vi "Hot Goal Detection - Image Compare.vi"(0 "Image In":T1, 7 "error in":errorcluster) -> (20 "Image Out":T1, 21 "Matches (tape)":T2(array[cluster]) {"Bounding Box"."y" format="%.2f"; "Bounding Box"."x" format="%.2f"; "Position"."y" format="%.2f"; "Position"."x" format="%.2f"; "Score" format="%.2f"; "Scale" format="%.2f"; "Angle" format="%.2f"}, 27 "error out":errorcluster)   [LabVIEW 2013]
uses:
  <vilib>/vision/Image Controls.llb/IMAQ Image.ctl
  <vilib>/vision/NI_Vision_Development_Module.lvlib
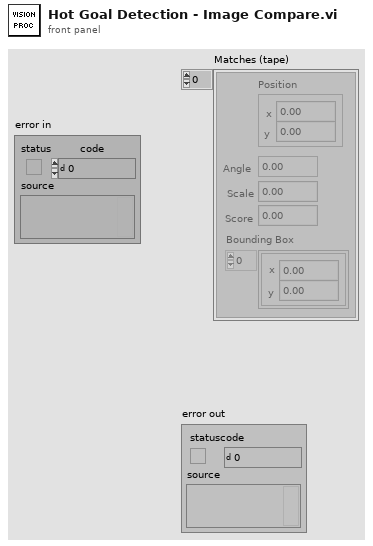
[diagram p1: front panel]
types:
  T1 = typedef "IMAQ Image.ctl" = refnum<image>
  T2 = cluster{"Position":cluster{"x":sgl, "y":sgl}, "Angle":sgl, "Scale":sgl, "Score":sgl, "Bounding Box":cluster{"x":sgl, "y":sgl}[]}[]
  T3 = typedef "Image Type" = u32
  T4 = cluster{"Global Rectangle":i32[], "Contours":cluster{"ID":enum32{"External", "Internal"}, "Type":u32, "Coordinates":i32[]}[]}
  T5 = cluster{"Brightness":sgl, "Contrast":sgl, "Gamma":sgl}
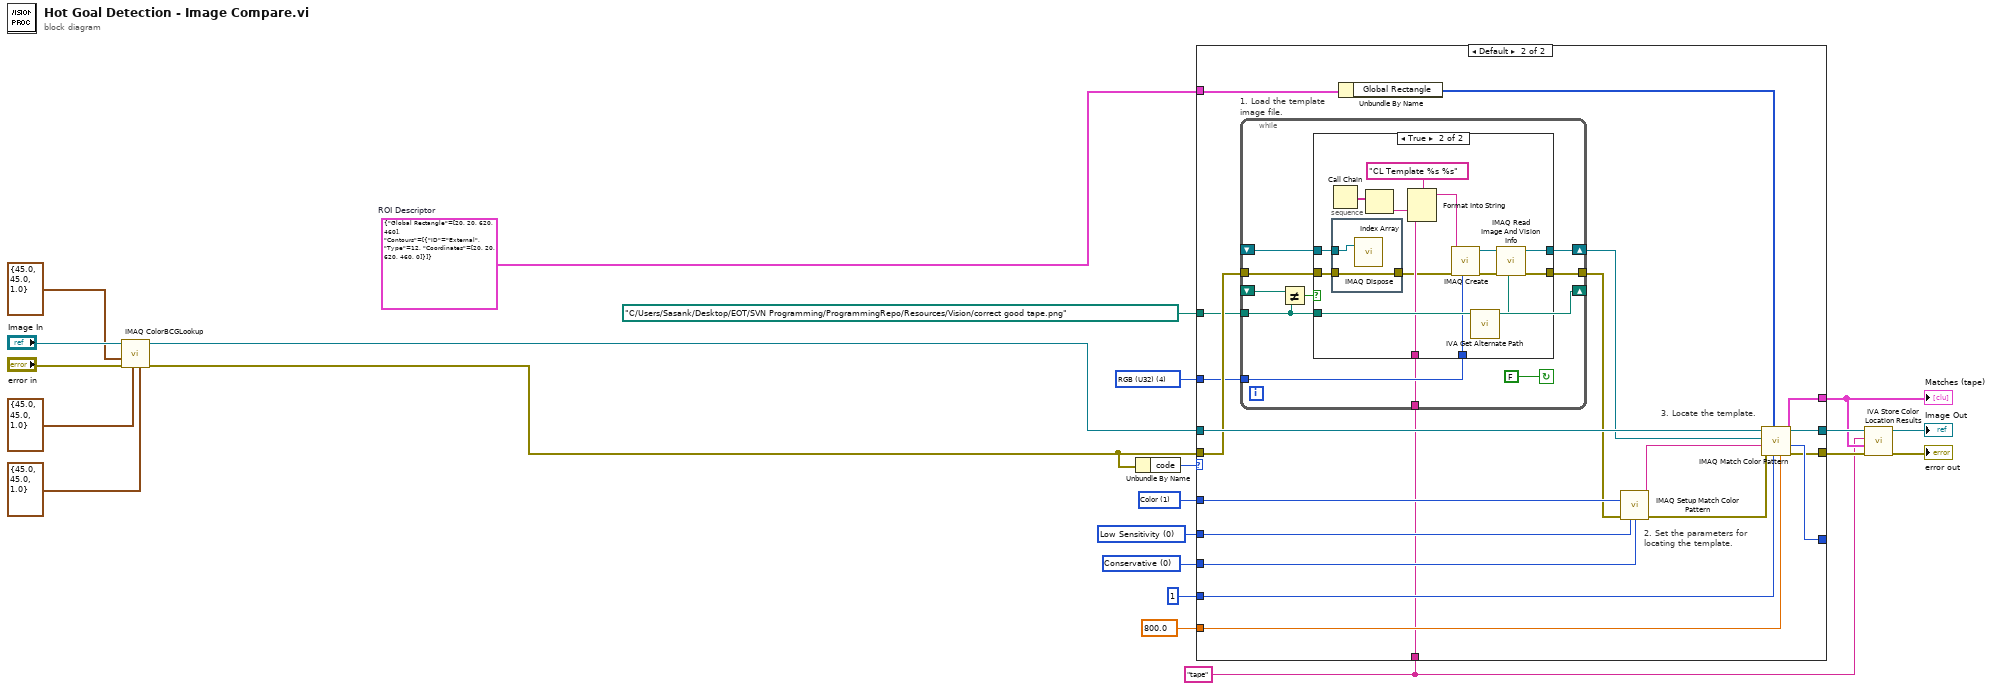
[diagram p0: block diagram]
diagram:
  w1 = "tape" ("Step Name")
  w10 = T3 4 items=["Grayscale (U8)", "Grayscale (I16)", "Grayscale (SGL)", "Complex (CSG)", "RGB (U32)", "HSL (U32)", "RGB (U64)"] ("Image Type")
  w12 = u32 0 items=["Conservative", "Balance", "Aggressive", "Very Aggressive"] ("Search Strategy")
  w13 = u32 0 items=["Low Sensitivity", "Medium Sensitivity", "High Sensitivity"] ("Color Sensitivity")
  w14 = u32 1 items=["Color and Shape", "Color", "Shape"] ("Match Feature Mode")
  w9 = T4 {"Global Rectangle"=[20, 20, 620, 460], "Contours"=[{"ID"=enum."External", "Type"=12, "Coordinates"=[20, 20, 620, 460, 0]}]}  # ROI Descriptor
  n1 = call "IMAQ ColorBCGLookup"("Blue BCG Values"=T5 {"Brightness"=45.0, "Contrast"=45.0, "Gamma"=1.0}, "Green BCG Values"=T5 {"Brightness"=45.0, "Contrast"=45.0, "Gamma"=1.0}, "error in (no error)"="error in", "Red BCG Values"=T5 {"Brightness"=45.0, "Contrast"=45.0, "Gamma"=1.0}, "Image Src"="Image In") -> ("error out"=w20:errorcluster, "Image Dst Out"=w8:T1)  [unwired: 2 in, 3 out]
  n2 = Unbundle By Name(w20) -> ("code"=w7:i32)
  n3 = case shown="Default" w7 {
    tunnel: sgl 800.0 ("Minimum Match Score") -> [_ w42]
    tunnel: 1 ("Number of Matches Requested") -> [_ w41]
    tunnel: [_ w40] -> _
    tunnel: w14 -> [_ w39]
    tunnel: w13 -> [_ w38]
    tunnel: w12 -> [_ w37]
    tunnel: path "C:/Users/Sasank/Desktop/EOT/SVN Programming/ProgrammingRepo/Resources/Vision/correct good tape.png" ("File Path") -> [_ w29]
    tunnel: w10 -> [_ w28]
    tunnel: w20 -> [_ w30]
    tunnel: w9 -> [_ w34]
    tunnel: [_ w32] -> w2
    tunnel: w8 -> [w23 w31]
    tunnel: [w23 w31] -> w3
    tunnel: [_ w25] -> w5
    tunnel: w1 -> [_ w24]
    frame -1074396199, -1074396198 {
      # "Discard Coordinate System Error"
    }
    frame Default {
      # "3. Locate the template."
      # "2. Set the parameters for\nlocating the template."
      n4 = while "1. Load the template image file." {
        shift-right: [w52] -> w27
        shift-left: _ -> [w51]
        tunnel: [w49] -> w26
        tunnel: w30 -> [w48]
        tunnel: w29 -> [w43]
        tunnel: w28 -> [w47]
        tunnel: w24 -> [w46]
        shift-right: [w43] -> _
        shift-left: _ -> [w45]
        stop <- FALSE continue-if-true
        n5 = Not Equal?(x=w45, y=w43) -> (x != y?=w44:bool)
        n6 = case shown="True" w44 {
          tunnel: [w54 w67] -> w52
          tunnel: w51 -> [w54 w59]
          tunnel: [w53 w64] -> w49
          tunnel: w48 -> [w53 w58]
          tunnel: w47 -> [_ w63]
          tunnel: w46 -> [_ w60]
          tunnel: w43 -> [_ w56]
          frame False {
          }
          frame True {
            n7 = Call Chain() -> (call chain=w62:string[])
            n8 = stacked-sequence {
              tunnel: w59 -> [w71]
              tunnel: w58 -> [w70]
              tunnel: [w70] -> w57
              frame #0 {
                n9 = call "IMAQ Dispose"("Image"=w71) -> ()  [unwired: 2 in, 4 out]
              }
            }
            n10 = Index Array(array=w62) -> (element=w61:string)  [unwired: 1 in]
            n11 = Format Into String(format string="CL Template %s %s" ("Image Name"), w61, w60) -> (resulting string=w69:string)  [unwired: 2 in, 1 out]
            n12 = call "IMAQ Create"("Image Name"=w69, "Image Type"=w63, "error in (no error)"=w57) -> ("New Image"=w66:T1, "error out"=w65:errorcluster)  [unwired: 1 in, 1 out]
            n13 = call <vilib>:"IVA Get Alternate Path.vi"("Path In"=w56) -> ("Path Out"=w55:path)  [unwired: 10 out]
            n14 = call "IMAQ Read Image And Vision Info"("File Path"=w55, "error in (no error)"=w65, "Image"=w66) -> ("error out"=w64:errorcluster, "Image Out"=w67:T1)  [unwired: 1 in, 6 out]
          }
        }
      }
      n15 = Unbundle By Name(w34) -> ("Global Rectangle"=w33:i32[])
      n16 = call "IMAQ Setup Match Color Pattern"("Match Feature Mode"=w39, "error in (no error)"=w26, "Color Sensitivity"=w38, "Search Strategy"=w37) -> ("Match Color Pattern Setup Data"=w36:string, "error out"=w35:errorcluster)  [unwired: 5 in, 5 out]
      n17 = call "IMAQ Match Color Pattern"("Minimum Match Score"=w42, "Number of Matches Requested"=w41, "Optional Rectangle"=w33, "error in (no error)"=w35, "Match Color Pattern Setup Data"=w36, "Template Image"=w27, "Image"=w31) -> ("error out"=w25:errorcluster, "Number of Matches"=w40:i32, "Matches"=w32:T2)  [unwired: 2 out]
    }
  }
  "Matches (tape)" <- w2
  n18 = call <vilib>:"IVA Store Color Location Results.vi"("error in (no error)"=w5, "Matches"=w2, "Step Name"=w1, "Image in"=w3) -> ("error out"=→"error out":errorcluster, "Image dup"=→"Image Out":T1)  [unwired: 6 out]
